vi "Test_Motor.vi"() -> ()   [LabVIEW 2014]
uses:
  <userlib>/UCSD Robotics Lab/Robotics-Cape/LV/libroboticscape.lvlib
panel:
  out "Voltage":sgl format="%#_4g"
  out "Battery Indicator":bool
  out "Timing Block":T1 {"Actual Hz" format="%#_3g"; "Dt" format="%#_4g"; "Average Hz" format="%#_4g"}
  out "Motor Cycle Count":dbl
  in  "On/Off":bool
  in  "duty":sgl=0.5 min=-1 max=1 step=0.05 format="%#_4g"
  in  "Motor":enum16{"All", "1", "2", "3", "4"}(ring)
  in  "Mode":T2(ring)
  out "State":T3(ring)
  in  "stop":bool
  # "Always stop the VI using the rectangular STOP button above, never with the round stopsign (Abort)"
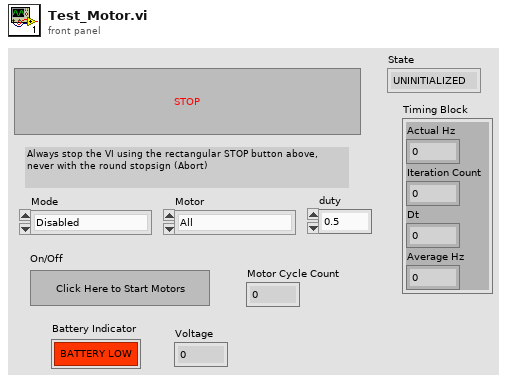
[diagram p1: front panel]
types:
  T1 = cluster{"Actual Hz":dbl, "Iteration Count":dbl, "Dt":dbl, "Average Hz":dbl}
  T2 = enum16{"Disabled", "Normal", "Brake", "Free", "Sweep"}
  T3 = enum16{"UNINITIALIZED", "RUNNING", "PAUSED", "EXITING"}
  T4 = enum16{"UNINITIALIZED", "RUNING", "PAUSED", "EXITING"}
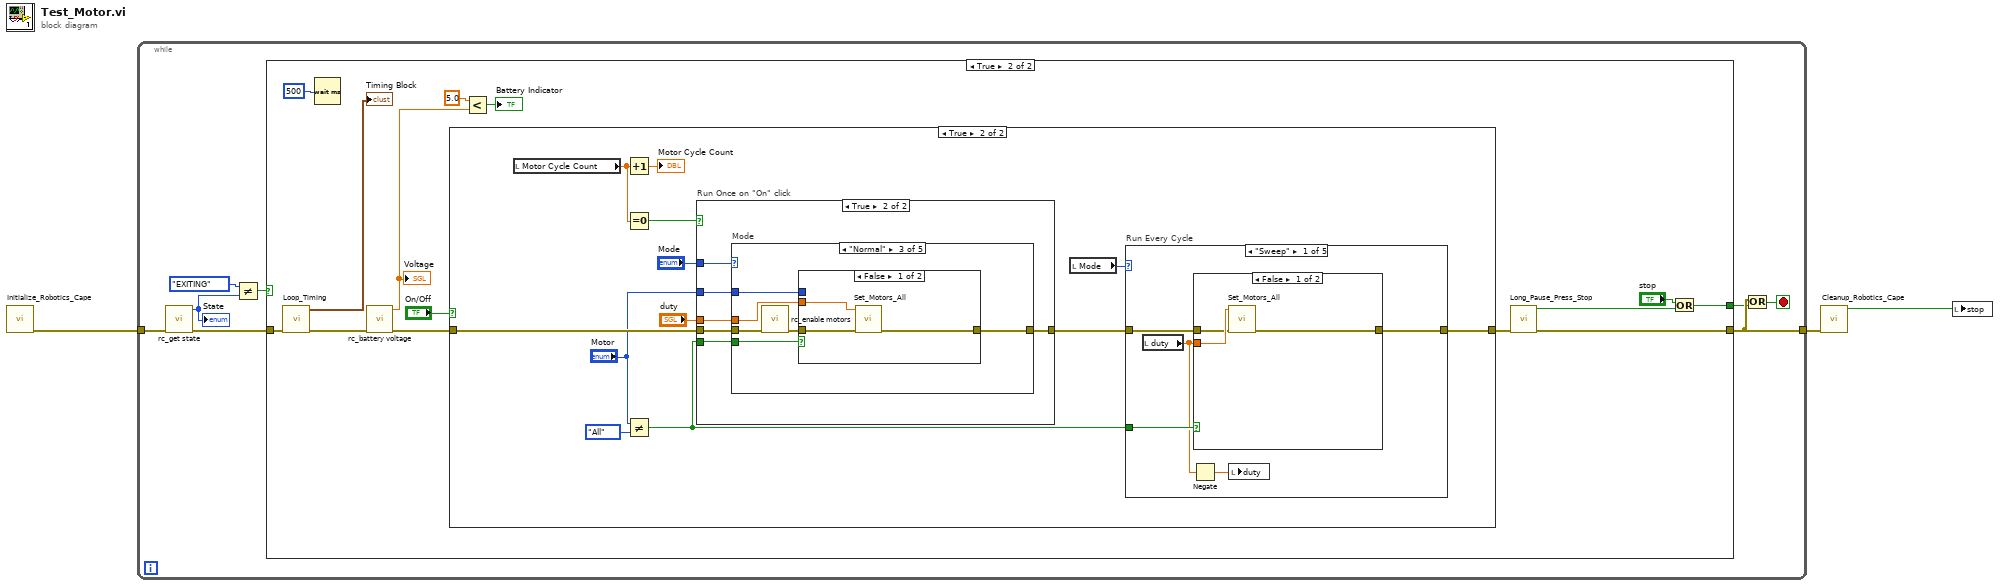
[diagram p0: block diagram]
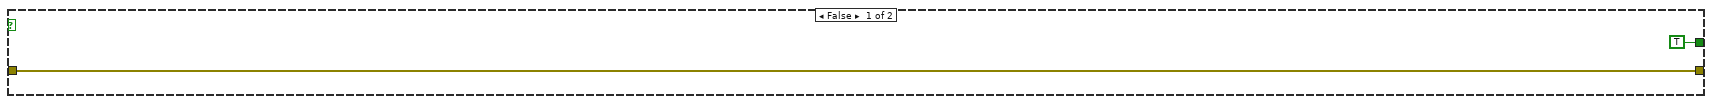
[diagram p2: hidden frame]
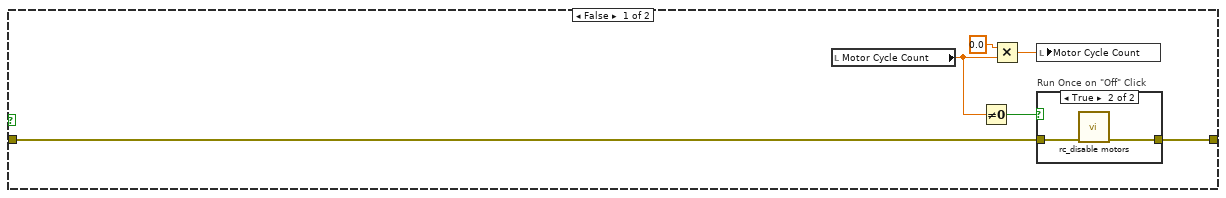
[diagram p3: hidden frame]
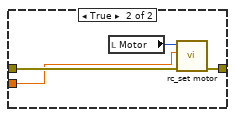
[diagram p5: hidden frame]
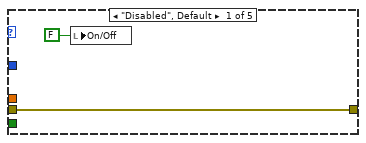
[diagram p11: hidden frame]
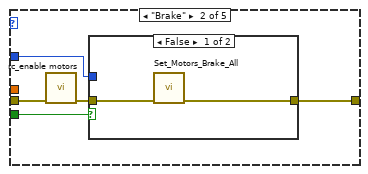
[diagram p12: hidden frame]
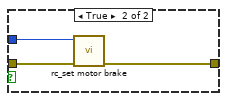
[diagram p13: hidden frame]
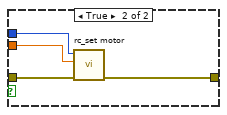
[diagram p14: hidden frame]
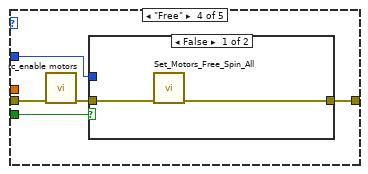
[diagram p15: hidden frame]
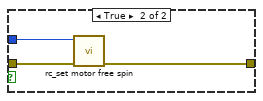
[diagram p16: hidden frame]
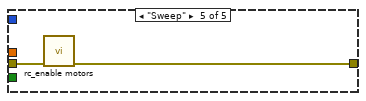
[diagram p17: hidden frame]
diagram:
  n1 = call "Initialize_Robotics_Cape.vi"() -> ("error out"=w2:errorcluster)  [unwired: 11 in]
  n2 = while {
    tunnel: w2 -> [w9]
    tunnel: [w11] -> w3
    stop <- w10 stop-if-true
    n3 = call <userlib>:"rc_get state.vi"("error in (no error)"=w9) -> ("error out"=w8:errorcluster, "function return"=w6:u32)  [unwired: 9 in]
    "State" <- w6
    n4 = Not Equal?(x=T4."EXITING" ("State 2"), y=w6) -> (x != y?=w5:bool)
    n5 = case shown="True" w5 {
      tunnel: [w13 w14] -> w11
      tunnel: w8 -> [w13 w25]
      tunnel: [TRUE w17] -> w4
      frame False {
      }
      frame True {
        n6 = call "Loop_Timing.vi"("error in"=w25) -> ("error out"=w23:errorcluster, "Timing Block"=→"Timing Block":T1)  [unwired: 9 in]
        n7 = Wait (ms)(milliseconds to wait=u32 500) -> ()  [unwired: 1 out]
        n8 = call <userlib>:"rc_battery voltage.vi"("error in (no error)"=w23) -> ("error out"=w22:errorcluster, "function return"=w21:sgl)  [unwired: 9 in]
        "Voltage" <- w21
        n9 = case shown="True" "On/Off" {
          tunnel: [w32 w38] -> w15
          tunnel: w22 -> [w33 w46]
          frame False {
            n10 = local read "Motor Cycle Count"() -> (w28:dbl)
            n11 = Not Equal To 0?(x=w28) -> (x != 0?=w29:bool)
            n12 = Multiply(x=0.0 ("On Count"), y=w28) -> (x*y=w31:dbl)
            n13 = local write "Motor Cycle Count"(w31) -> ()
            n14 = case "Run Once on \"Off\" Click" shown="True" w29 {
              tunnel: w33 -> [w34 w36]
              tunnel: [w34 w35] -> w32
              frame False {
              }
              frame True {
                n15 = call <userlib>:"rc_disable motors.vi"("error in (no error)"=w36) -> ("error out"=w35:errorcluster)  [unwired: 9 in, 1 out]
              }
            }
          }
          frame True {
            n16 = local read "Motor Cycle Count"() -> (w45:dbl)
            n17 = Increment(x=w45) -> (x+1=→"Motor Cycle Count":dbl)
            n18 = Equal To 0?(x=w45) -> (x = 0?=w44:bool)
            n19 = Not Equal?(x="Motor", y=enum16{"All", "1", "2", "3", "4"}."All" ("Motor 2")) -> (x != y?=w39:bool)
            n20 = case "Run Once on \"On\" click" shown="True" w44 {
              tunnel: w46 -> [w65 w70]
              tunnel: [w65 w71] -> w41
              tunnel: "Mode" -> [_ w69]
              tunnel: w39 -> [_ w68]
              tunnel: "duty" -> [_ w67]
              tunnel: "Motor" -> [_ w66]
              frame False {
              }
              frame True {
                n21 = case "Mode" shown="\"Normal\"" w69 {
                  tunnel: [w73 w78 w89 w101 w107] -> w71
                  tunnel: w70 -> [w73 w77 w88 w100 w108]
                  tunnel: w68 -> [_ w75 w86 w98 _]
                  tunnel: w67 -> [_ _ w85 _ _]
                  tunnel: w66 -> [_ w74 w84 w97 _]
                  frame "Disabled", Default {
                    n22 = local write "On/Off"(FALSE ("On/Off")) -> ()
                  }
                  frame "Brake" {
                    n23 = call <userlib>:"rc_enable motors.vi"("error in (no error)"=w77) -> ("error out"=w76:errorcluster)  [unwired: 9 in, 1 out]
                    n24 = case shown="False" w75 {
                      tunnel: [w79 w83] -> w78
                      tunnel: w76 -> [w80 w82]
                      tunnel: w74 -> [_ w81]
                      frame False {
                        n25 = call "Set_Motors_Brake_All.vi"("error in (no error)"=w80) -> ("error out"=w79:errorcluster)  [unwired: 10 in]
                      }
                      frame True {
                        n26 = call <userlib>:"rc_set motor brake.vi"("error in (no error)"=w82, "motor"=w81) -> ("error out"=w83:errorcluster)  [unwired: 8 in, 1 out]
                      }
                    }
                  }
                  frame "Normal" {
                    n27 = call <userlib>:"rc_enable motors.vi"("error in (no error)"=w88) -> ("error out"=w87:errorcluster)  [unwired: 9 in, 1 out]
                    n28 = case shown="False" w86 {
                      tunnel: [w91 w96] -> w89
                      tunnel: w87 -> [w92 w95]
                      tunnel: w85 -> [w90 w94]
                      tunnel: w84 -> [_ w93]
                      frame False {
                        n29 = call "Set_Motors_All.vi"("error in (no error)"=w92, "duty"=w90) -> ("error out"=w91:errorcluster)  [unwired: 9 in]
                      }
                      frame True {
                        n30 = call <userlib>:"rc_set motor.vi"("error in (no error)"=w95, "duty"=w94, "motor"=w93) -> ("error out"=w96:errorcluster)  [unwired: 7 in, 1 out]
                      }
                    }
                  }
                  frame "Free" {
                    n31 = call <userlib>:"rc_enable motors.vi"("error in (no error)"=w100) -> ("error out"=w99:errorcluster)  [unwired: 9 in, 1 out]
                    n32 = case shown="False" w98 {
                      tunnel: [w102 w106] -> w101
                      tunnel: w99 -> [w103 w105]
                      tunnel: w97 -> [_ w104]
                      frame False {
                        n33 = call "Set_Motors_Free_Spin_All.vi"("error in (no error)"=w103) -> ("error out"=w102:errorcluster)  [unwired: 10 in]
                      }
                      frame True {
                        n34 = call <userlib>:"rc_set motor free spin.vi"("error in (no error)"=w105, "motor"=w104) -> ("error out"=w106:errorcluster)  [unwired: 8 in, 1 out]
                      }
                    }
                  }
                  frame "Sweep" {
                    n35 = call <userlib>:"rc_enable motors.vi"("error in (no error)"=w108) -> ("error out"=w107:errorcluster)  [unwired: 9 in, 1 out]
                  }
                }
              }
            }
            n36 = local read "Mode"() -> (w37:T2)
            n37 = case "Run Every Cycle" shown="\"Sweep\"" w37 {
              tunnel: w41 -> [w53 w61 w62 w63 w64]
              tunnel: w39 -> [w52 _ _ _ _]
              tunnel: [w51 w61 w62 w63 w64] -> w38
              frame "Sweep" {
                n38 = local read "duty"() -> (w50:sgl)
                n39 = Negate(x=w50) -> (-x=w49:sgl)
                n40 = case shown="False" w52 {
                  tunnel: [w54 w60] -> w51
                  tunnel: w53 -> [w55 w59]
                  tunnel: w50 -> [w56 w58]
                  frame False {
                    n41 = call "Set_Motors_All.vi"("error in (no error)"=w55, "duty"=w56) -> ("error out"=w54:errorcluster)  [unwired: 9 in]
                  }
                  frame True {
                    n42 = local read "Motor"() -> (w57:enum16{"All", "1", "2", "3", "4"})
                    n43 = call <userlib>:"rc_set motor.vi"("error in (no error)"=w59, "duty"=w58, "motor"=w57) -> ("error out"=w60:errorcluster)  [unwired: 7 in, 1 out]
                  }
                }
                n44 = local write "duty"(w49) -> ()
              }
              frame "Free" {
              }
              frame "Brake" {
              }
              frame "Normal" {
              }
              frame "Disabled", Default {
              }
            }
          }
        }
        n45 = Less?(x=sgl 5.0, y=w21) -> (x < y?=→"Battery Indicator":bool)
        n46 = call "Long_Pause_Press_Stop.vi"("error in (no error)"=w15) -> ("error out"=w14:errorcluster, "Stop"=w16:bool)  [unwired: 9 in]
        n47 = Or(x="stop", y=w16) -> (x .or. y?=w17:bool)
      }
    }
    n48 = Or(x=w11, y=w4) -> (x .or. y?=w10:bool)
  }
  n49 = call "Cleanup_Robotics_Cape.vi"("error in (no error)"=w3) -> ("Stop Local Variabl"=w1:bool)  [unwired: 9 in, 1 out]
  n50 = local write "stop"(w1) -> ()
